vi "test_Create Response.vi"(8 "error in (no error)":errorcluster, 11 "TestCase in":refnum<class "Instrument Addon Scripting API Messages Unit Tests.lvclass">) -> (0 "error out":errorcluster, 3 "TestCase out":refnum<class "Instrument Addon Scripting API Messages Unit Tests.lvclass">)   [LabVIEW 2019, in "Instrument Addon Scripting API Messages Unit Tests.lvclass"]
uses:
  Instrument Addon Scripting API Messages Unit Tests.lvclass
  Instrument Addon Scripting API Messages Unit Tests.lvclass/Instrument Addon Scripting API Messages Unit Tests.ctl
  Addon/Addon Shared/SubVIs/Constants.vi
  <vilib>/NI/NI VeriStand Advanced SysDef API/_SubVIs/SysDef.Search.GUID.vi
  <vilib>/addons/_JKI Toolkits/VI Tester/TestCase.llb/TestCase.lvclass
  Instrument Addon Scripting API Test Assets/Instrument Addon Scripting API Test Assets.lvclass
  <vilib>/NI/NI VeriStand Advanced SysDef API/SysDef API/Advanced System Definition.lvlib
  Addon/Addon Shared/Instrument Addon Shared.lvlib
  APIs/Scripting API/Instrument Addon Scripting API.lvlib
  C:/Program Files (x86)/National Instruments/LabVIEW 2019/vi.lib/addons/_JKI Toolkits/VI Tester/TestCase.llb/TestCase.lvclass
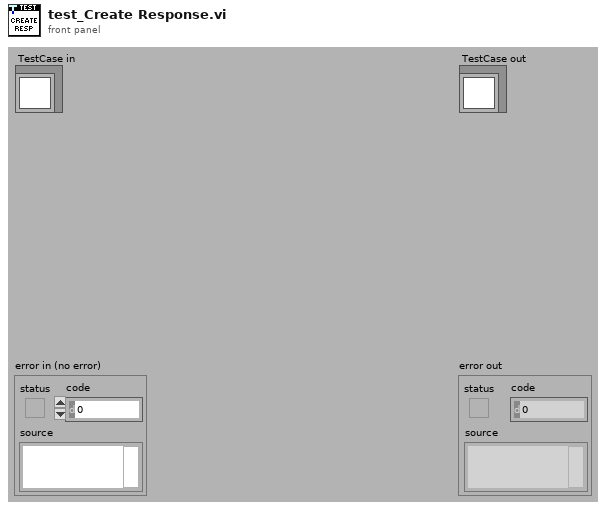
[diagram p1: front panel]
types:
  T1 = typedef "Custom Device API.lvlib/Custom Device Item Ref.ctl" = u64
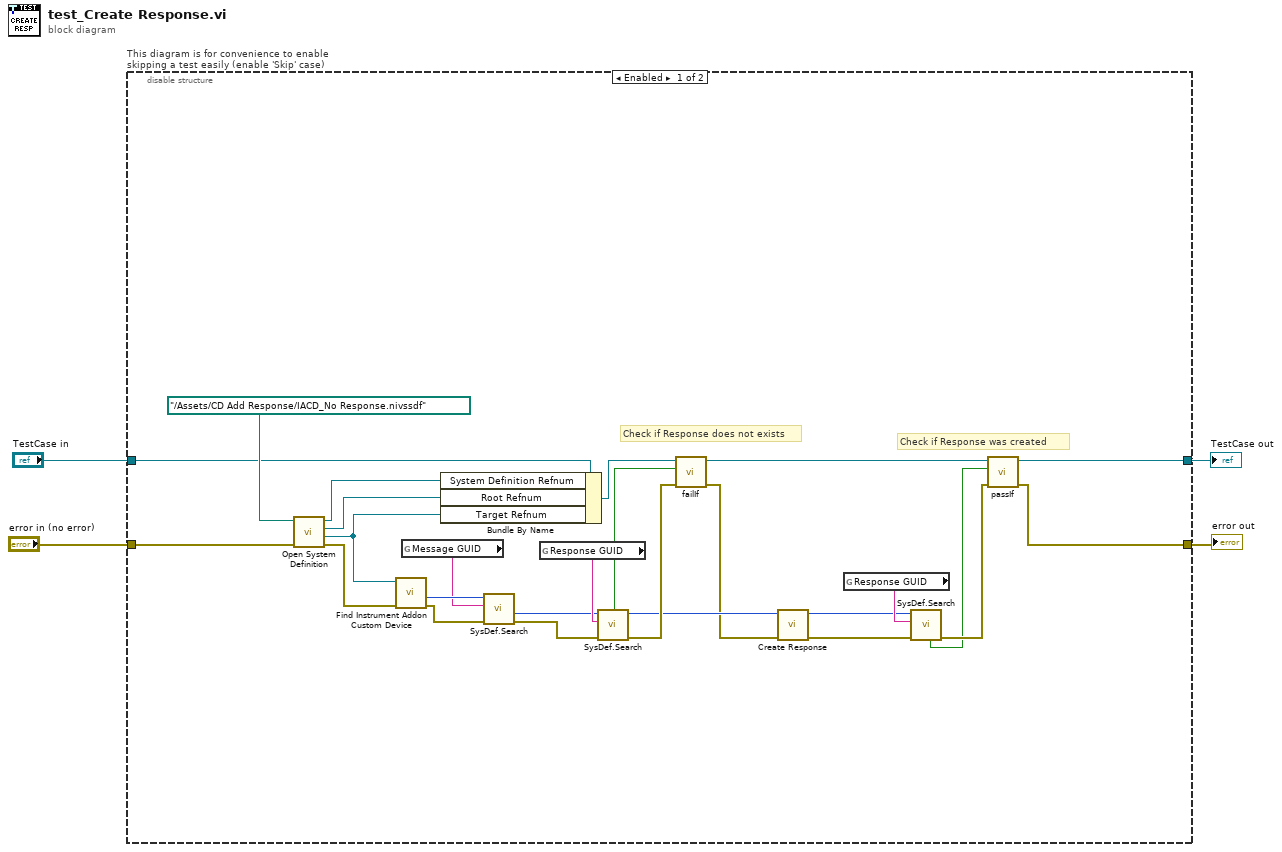
[diagram p0: block diagram]
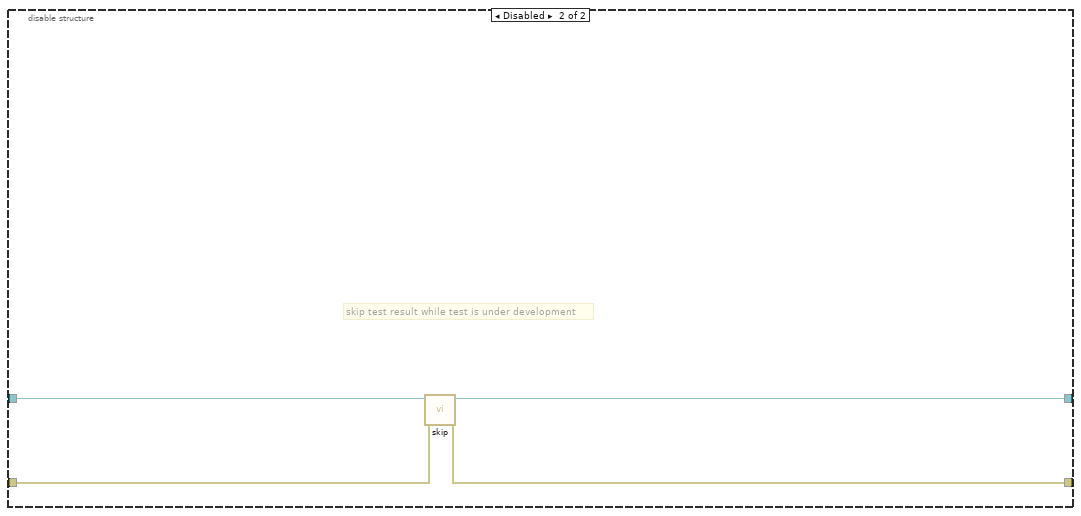
[diagram p2: hidden frame]
diagram:
  n1 = disable-structure "This diagram is for convenience to enable skipping a test easily (enable 'Skip' case)" shown="Enabled" {
    disable-tunnel: "TestCase in" -> [w13 w34]
    disable-tunnel: [w19 w32] -> w1
    disable-tunnel: [w20 w33] -> w3
    disable-tunnel: "error in (no error)" -> [w29 w31]
    frame Enabled {
      # "Check if Response was created"
      # "Check if Response does not exists"
      n2 = call "Open System Definition.vi"("error in (no error)"=w29, "System Definition File"=path "../Assets/CD Add Response/IACD_No Response.nivssdf" ("SDF file")) -> ("error out"=w28:errorcluster, "Target Refnum"=w12:refnum<k24>, "Root Refnum"=w11:refnum<k24>, "System Definition Refnum"=w10:refnum<k24>)  [unwired: 6 in]
      n3 = call "Find Instrument Addon Custom Device.vi"("error in"=w28, "target in"=w12) -> ("error out"=w17:errorcluster, "NodeID"=w18:u64)  [unwired: 7 in, 1 out]
      n4 = global read "Constants.vi" "Message GUID"() -> (w16:string)
      n5 = Bundle By Name(cluster=w13, "System Definition Refnum"=w10, "Root Refnum"=w11, "Target Refnum"=w12) -> (w9:refnum<class "Instrument Addon Scripting API Messages Unit Tests.lvclass">)
      n6 = call-poly <vilib>:"SysDef.Search.vi"("error in (no error)"=w17, "GUID"=w16, "nodeID"=w18) -> ("error out"=w15:errorcluster, "Value out"=w14:u64)  [unwired: 5 in, 2 out]
      n7 = global read "Constants.vi" "Response GUID"() -> (w26:string)
      n8 = call-poly <vilib>:"SysDef.Search.vi"("error in (no error)"=w15, "GUID"=w26, "nodeID"=w14) -> ("error out"=w24:errorcluster, "nodeID out"=w8:u64, "Found?"=w25:bool)  [unwired: 5 in, 1 out]
      n9 = call-dynamic "failIf.vi"("error in (no error)"=w24, "fail"=w25, "TestCase in"=w9) -> ("error out"=w7:errorcluster, "TestCase out"=w23:refnum<class "Instrument Addon Scripting API Messages Unit Tests.lvclass">)  [unwired: 7 in]
      n10 = call "Create Response.vi"("error in (no error)"=w7, "message refnum in"=w8) -> ("error out"=w6:errorcluster, "message refnum out"=w5:T1)  [unwired: 7 in, 1 out]
      n11 = global read "Constants.vi" "Response GUID"() -> (w27:string)
      n12 = call-poly <vilib>:"SysDef.Search.vi"("error in (no error)"=w6, "GUID"=w27, "nodeID"=w5) -> ("error out"=w22:errorcluster, "Found?"=w21:bool)  [unwired: 5 in, 2 out]
      n13 = call-dynamic "passIf.vi"("error in (no error)"=w22, "pass"=w21, "TestCase in"=w23) -> ("error out"=w20:errorcluster, "TestCase out"=w19:refnum<class "Instrument Addon Scripting API Messages Unit Tests.lvclass">)  [unwired: 7 in]
    }
    frame Disabled {
      # "skip test result while test is under development"
      n14 = call <vilib>:"skip.vi"("error in (no error)"=w31, "TestCase in"=w34) -> ("error out"=w33:errorcluster, "TestCase out"=w32:refnum<class "Instrument Addon Scripting API Messages Unit Tests.lvclass">)  [unwired: 8 in]
    }
  }
  "error out" <- w3
  "TestCase out" <- w1
